vi "DEMO_APD.vi"(8 "error in":errorcluster, 11 "command":string) -> (0 "error out":errorcluster, 3 "data ref":refnum<data-value>)   [LabVIEW 2010]
panel:
  in  "front panel VI Refnum":refnum<vi>
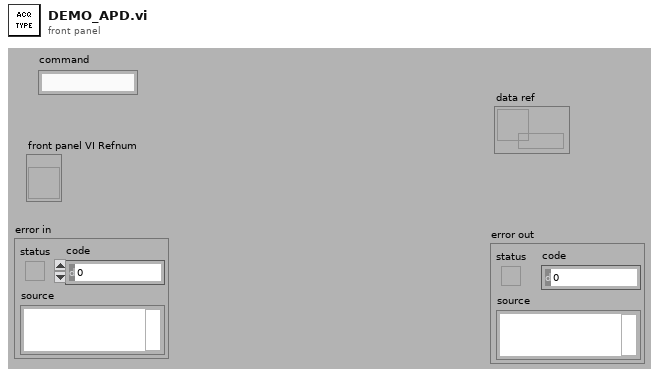
[diagram p1: front panel]
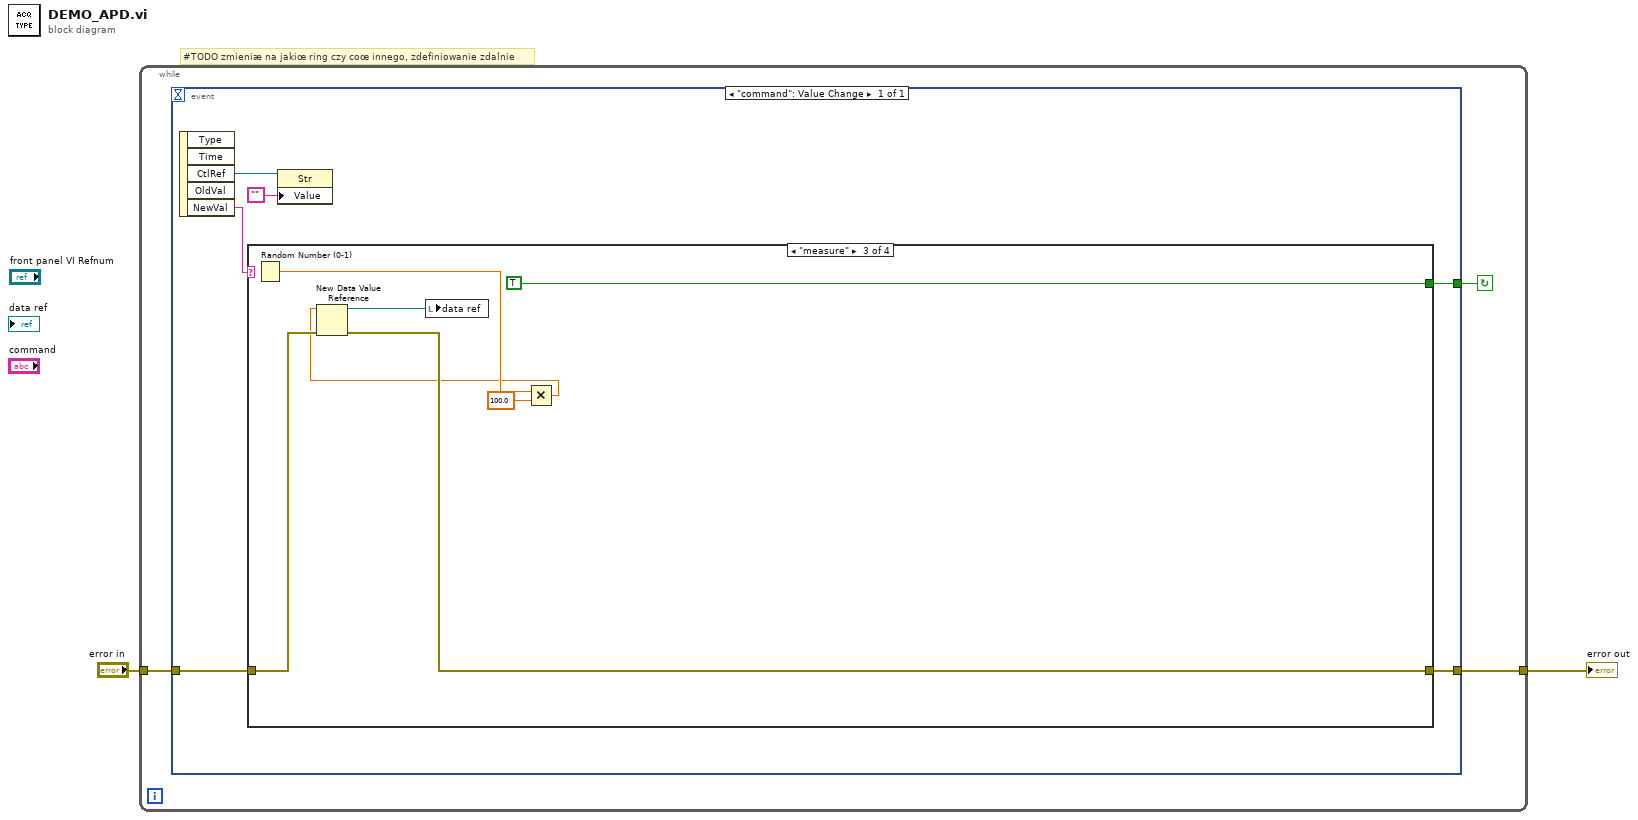
[diagram p0: block diagram]
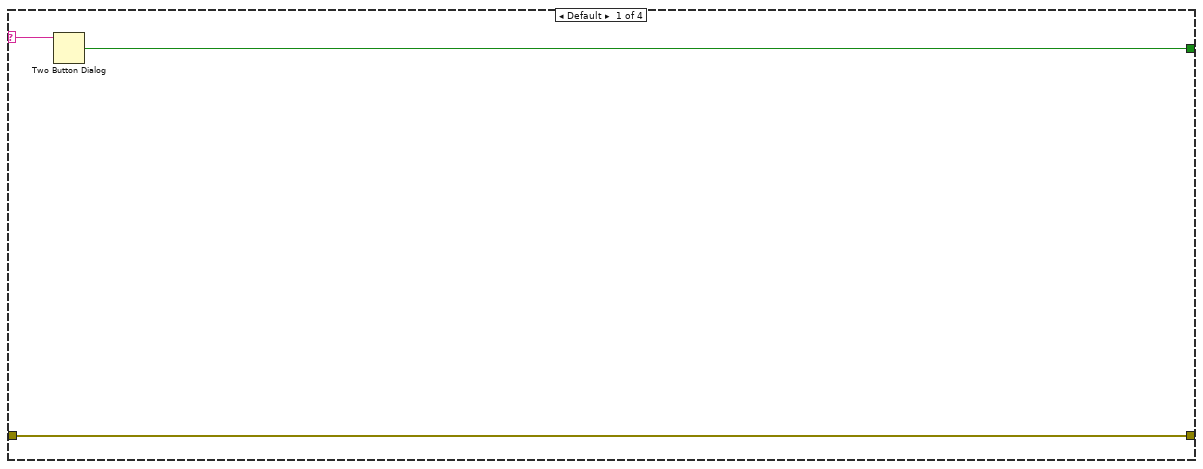
[diagram p2: hidden frame]
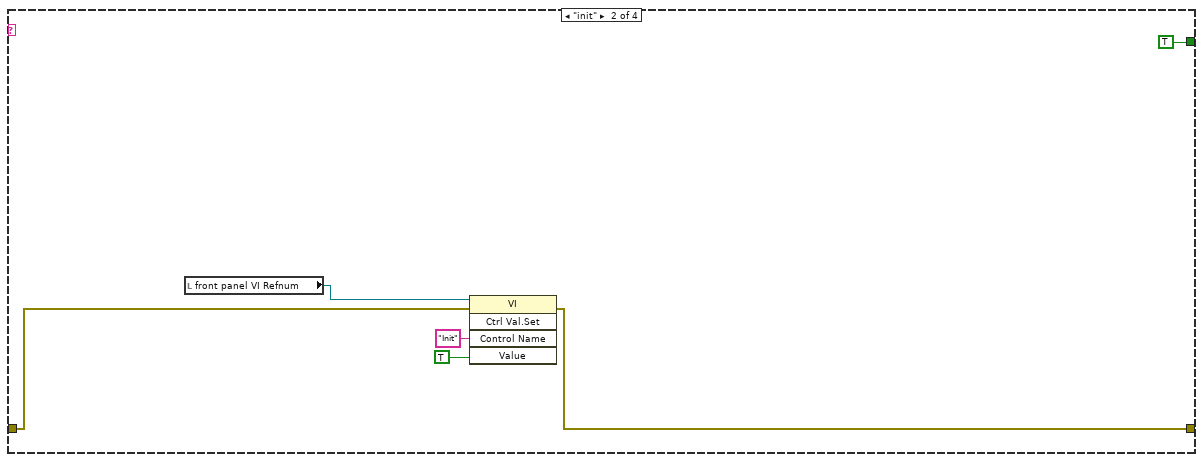
[diagram p3: hidden frame]
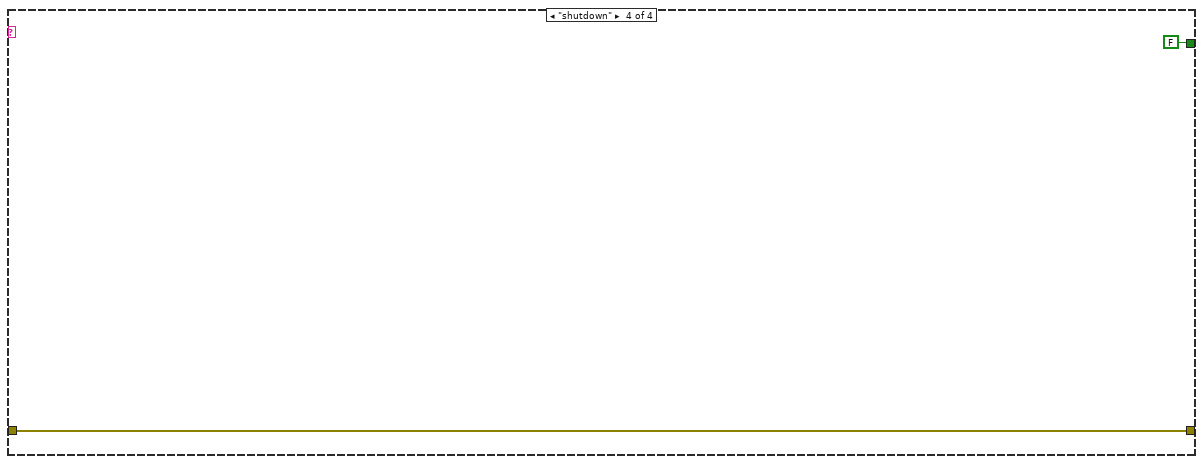
[diagram p4: hidden frame]
diagram:
  # "#TODO zmieniæ na jakiœ ring czy coœ innego, zdefiniowanie zdalnie"
  n1 = while {
    tunnel: [w3] -> w2
    tunnel: "error in" -> [w4]
    stop <- w5 continue-if-true
    n2 = event shown="[0] \"command\": Value Change" {
      selector: _ -> [_]
      dyn-events: _ -> [_]
      timeout: _ -> [_]
      tunnel: [w8] -> w5
      tunnel: w4 -> [w7]
      tunnel: [w6] -> w3
      event "command": Value Change {
        n3 = event-data() -> ("CtlRef"=w11:refnum<vi>, "NewVal"=w9:string)  [unwired: 1 in, 3 out]
        n4 = case shown="\"measure\"" w9 {
          selector: w9 -> [w14 _ _ _]
          tunnel: [w13 TRUE TRUE ("T button?") FALSE] -> w8
          tunnel: w7 -> [w12 w19 w25 w28]
          tunnel: [w12 w18 w24 w28] -> w6
          frame Default {
            n5 = Two Button Dialog(message=w14) -> (T button?=w13:bool)  [unwired: 2 in]
          }
          frame "init" {
            n6 = local read "front panel VI Refnum"() -> (w20:refnum<vi>)
            n7 = invoke class="VI" method="Ctrl Val.Set"(reference=w20, error in=w19, "Control Name"="Init", "Value"=TRUE) -> (error out=w18:errorcluster)  [unwired: 1 in, 4 out]
          }
          frame "measure" {
            n8 = Random Number (0-1)() -> (number: 0 to 1=w23:dbl)
            n9 = Multiply(x=w23, y=100.0) -> (x*y=w21:dbl)
            n10 = New Data Value Reference(data value=w21, error in=w25) -> (data value reference=w26:refnum<data-value>, error out=w24:errorcluster)
            n11 = local write "data ref"(w26) -> ()
          }
          frame "shutdown" {
          }
        }
        n12 = property class="Str"(reference=w11, "Value"="") -> ()  [unwired: 1 in, 2 out]
      }
    }
  }
  "error out" <- w2
